vi "Analog Output Engine.vi"(5 "Main Engine Q":refnum<queue>, 7 "TCP Enigine Q":refnum<queue>, 8 "error in":errorcluster, 10 "Engine Name":string, 11 "Varient Data":variant) -> (0 "error out":errorcluster)   [LabVIEW 2024]
doc: "All Rights Reserved © 2017 SyncSols"
uses:
  Controls/Analog Output SM Data Cluster.ctl
  Controls/AIO Command Q Cluster.ctl
  Controls/AO Interface Data Cluster.ctl
  Controls/AO Channel Configuration Cluster.ctl
  Controls/AO Timing Cluster.ctl
  Main Engine/Controls/Main Engine JSON Command State.ctl
  TCP Engine/Controls/TCP Engine I&O  Interupt Cluster.ctl
  Controls/Analog Output SM Cases.ctl
  Main Engine/Controls/Main Engine Engine No.Options.ctl
  Controls/AO JSON Data Cluster.ctl
  Main Engine/Controls/Main Engine Config Confirmation Cluster.ctl
  <vilib>/DAQmx/write.llb/DAQmx Write (Analog 1D Wfm NChan NSamp).vi
  <vilib>/DAQmx/create/channels.llb/DAQmx Create Channel (AO-Voltage-Basic).vi
  <vilib>/DAQmx/create/channels.llb/DAQmx Create Channel (AO-Current-Basic).vi
  <vilib>/DAQmx/configure/timing.llb/DAQmx Timing (Sample Clock).vi
  <vilib>/DAQmx/miscellaneous.llb/DAQmx Fill In Error Info.vi
  TCP Engine/TCP Engine.lvlib
  <resource>/objmgr/daqmx.rc
panel:
  in  "Data Cluster":T1={"Main Engine Respons  Q"=refnum, "TCP Engine Response Q"=refnum, "Start Notifier"=refnum, "Stop Notifier"=refnum, "AO Task"="", "Varient Data"=variant(string ""), "Engine Name"="", "Continous Data Generation"=FALSE, " Command Q"=refnum, "Interupt Q"=refnum, "AO Timing"={"samples per channel"=1000, "sample mode"=10178, "Sampling Rate"=1000.0}, "Configuration Data"=[], "Channel names"=[], "6738 Card?"=FALSE, "AO Log File Path"=path ""} {"AO Timing"."sample mode" items=["Finite Samples"=10178, "Continuous Samples"=10123, "Hardware Timed Single Point"=12522]}
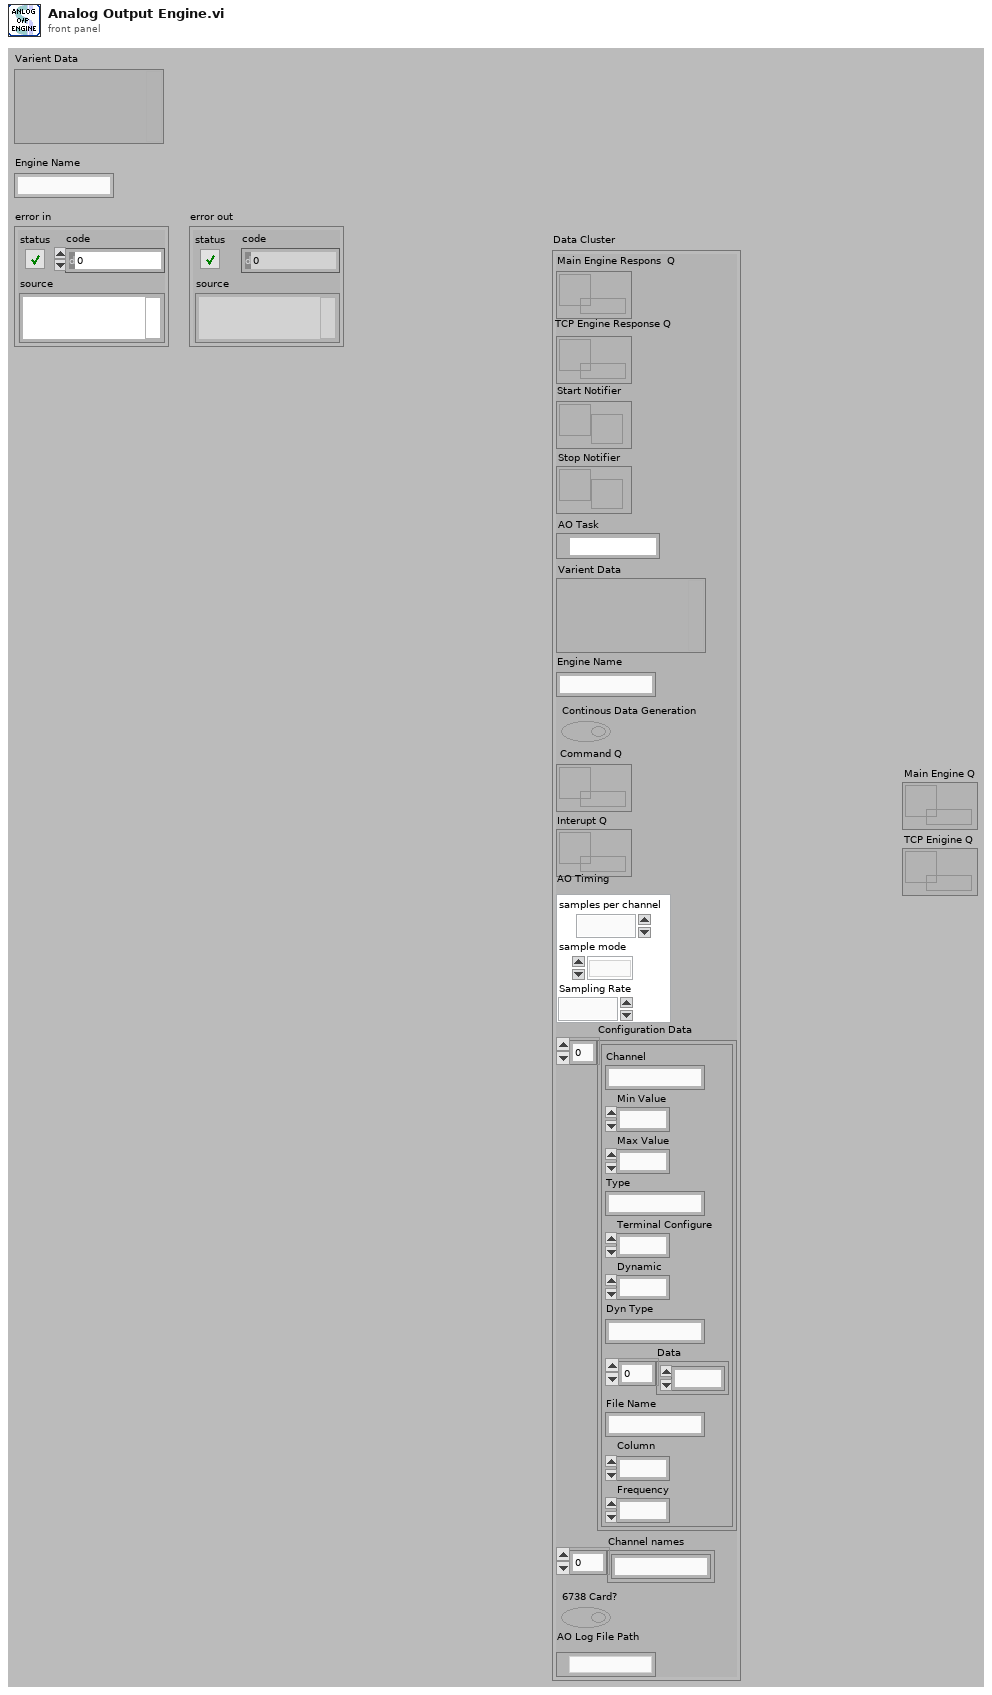
[diagram p1: front panel]
types:
  T1 = typedef "Analog Output SM Data Cluster.ctl" = cluster{"Main Engine Respons  Q":refnum<queue>, "TCP Engine Response Q":refnum<queue>, "Start Notifier":refnum<notifier>, "Stop Notifier":refnum<notifier>, "AO Task":refnum<k21>, "Varient Data":variant, "Engine Name":string, "Continous Data Generation":bool, " Command Q":refnum<queue>, "Interupt Q":refnum<queue>, "AO Timing":T2, "Configuration Data":T3[], "Channel names":string[], "6738 Card?":bool, "AO Log File Path":path}
  T2 = typedef "AO Timing Cluster.ctl" = cluster{"samples per channel":i32, "sample mode":i32, "Sampling Rate":dbl}
  T3 = typedef "AO Channel Configuration Cluster.ctl" = cluster{"Channel":string, "Min Value":dbl, "Max Value":dbl, "Type":string, "Terminal Configure":u16, "Dynamic":u8, "Dyn Type":string, "Data":dbl[], "File Name":string, "Column":i32, "Frequency":dbl}
  T4 = typedef "Analog Output SM Cases.ctl" = enum16{">Poll", ".........State Machine.........", ">Init", ">Error", ">Exit", "..........Analog Output..........", ">JSON to LV Data", ">Gen Dyn Data", ">Get Command", ">Configure", ">Start", ">Generate", ">Stop"}
  T5 = typedef "TCP Engine.lvlib/TCP Engine I&O  Interupt Cluster.ctl" = cluster{" Stop":bool, "JSON Variant":variant}
  T6 = typedef "AIO Command Q Cluster.ctl" = cluster{"Interface":string, "Interface Data":T7, "Command State":T8}
  T7 = typedef "AO Interface Data Cluster.ctl" = cluster{"Command":string, "SubCmd":string, "Data":T3[], "Timing":T2}
  T8 = typedef "Main Engine JSON Command State.ctl" = enum16{"Configure", "Start", "Exit"}
  T9 = typedef "Main Engine Engine No.Options.ctl" = enum16{"Init", "Update", "Response", "Get"}
  T10 = typedef "AO JSON Data Cluster.ctl" = cluster{"Interface":string, "Interface Data":T7}
  T11 = typedef "Main Engine Config Confirmation Cluster.ctl" = cluster{"Command":string, "Interface":string, "Status":string, "Board":string}
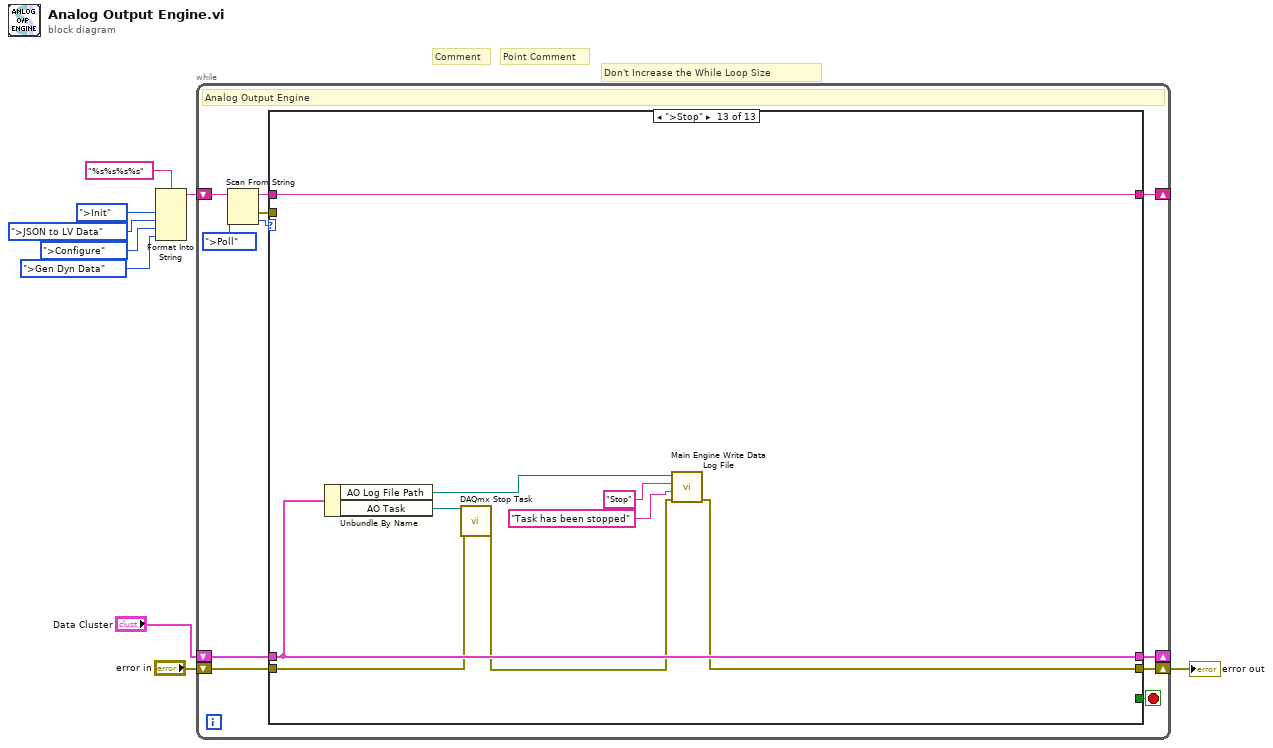
[diagram p0: block diagram]
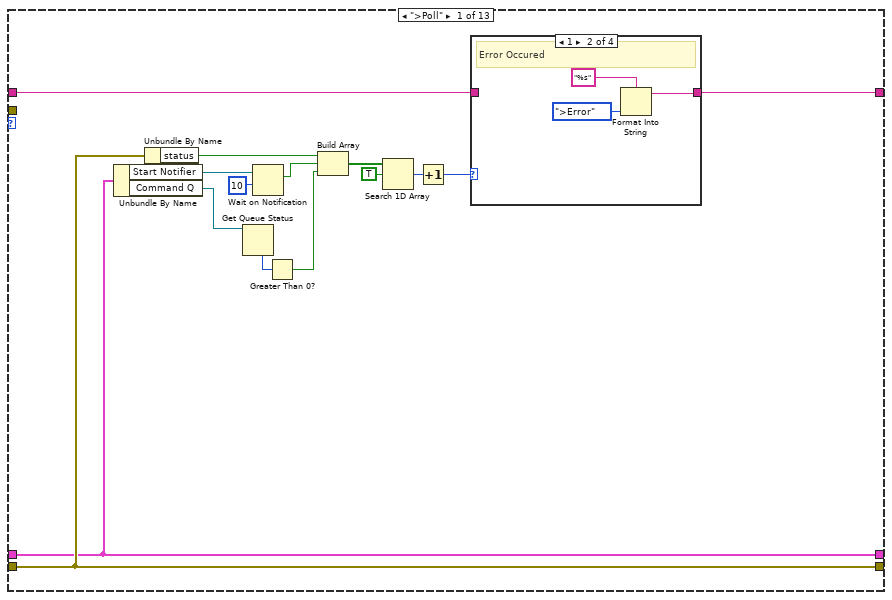
[diagram p2: hidden frame]
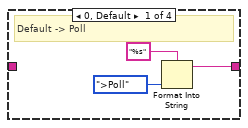
[diagram p3: hidden frame]
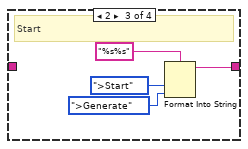
[diagram p4: hidden frame]
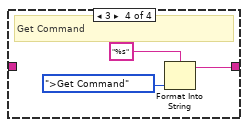
[diagram p5: hidden frame]
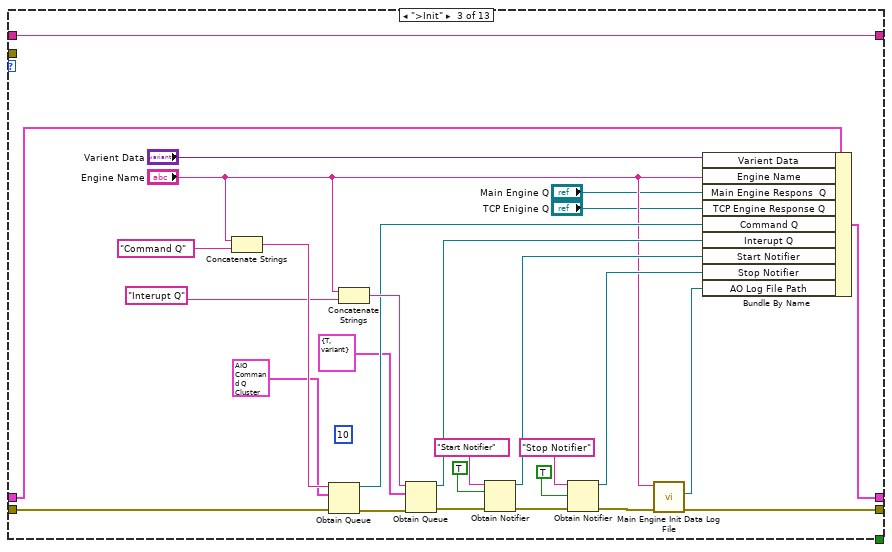
[diagram p7: hidden frame]
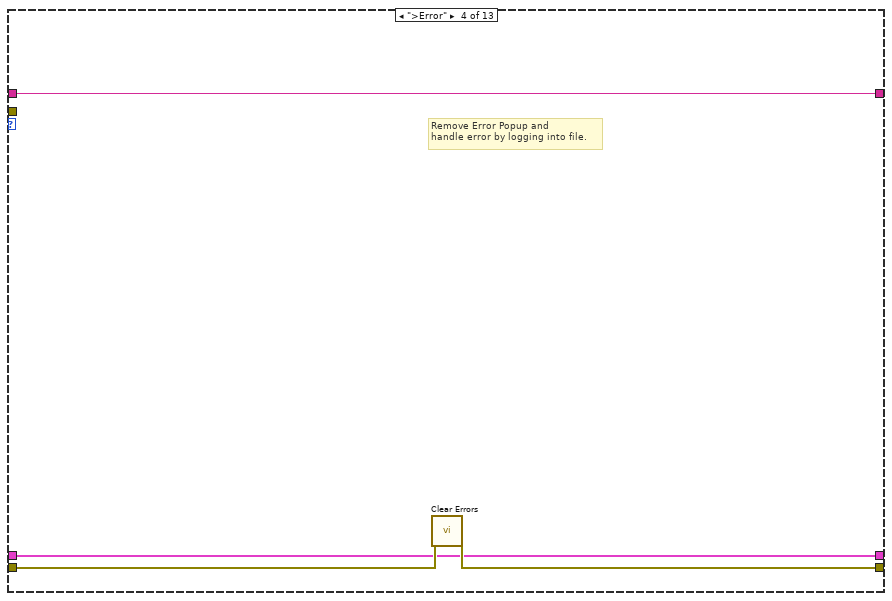
[diagram p8: hidden frame]
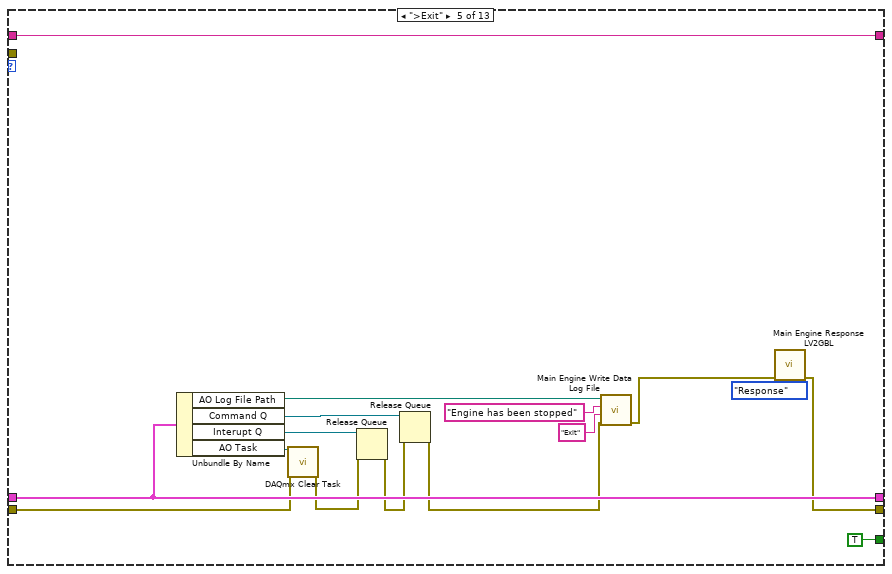
[diagram p9: hidden frame]
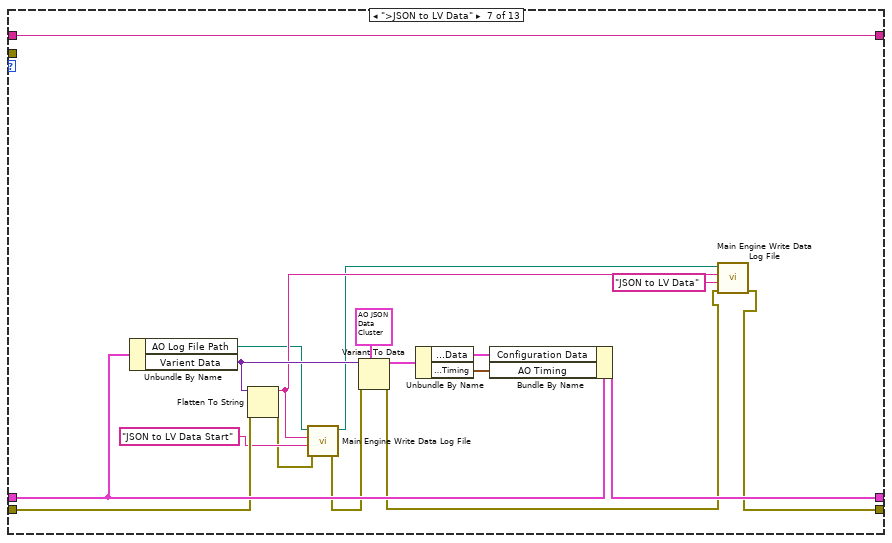
[diagram p11: hidden frame]
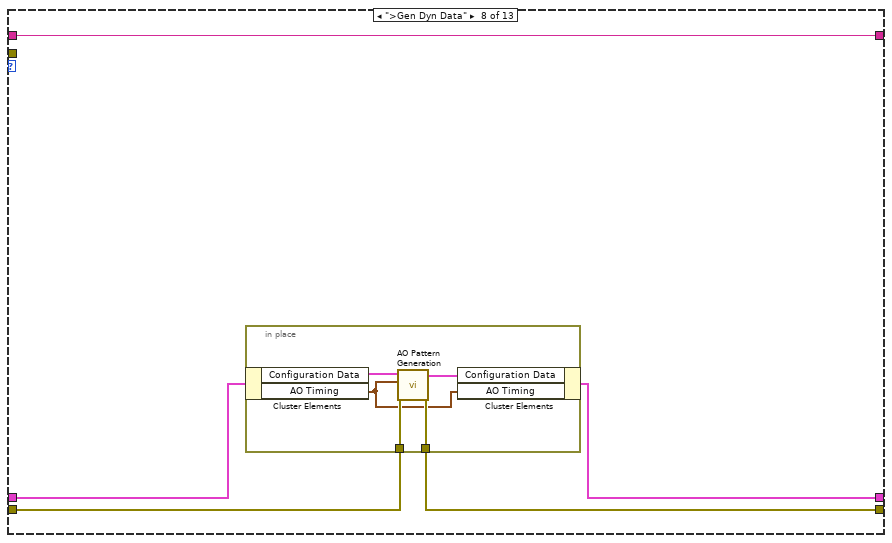
[diagram p12: hidden frame]
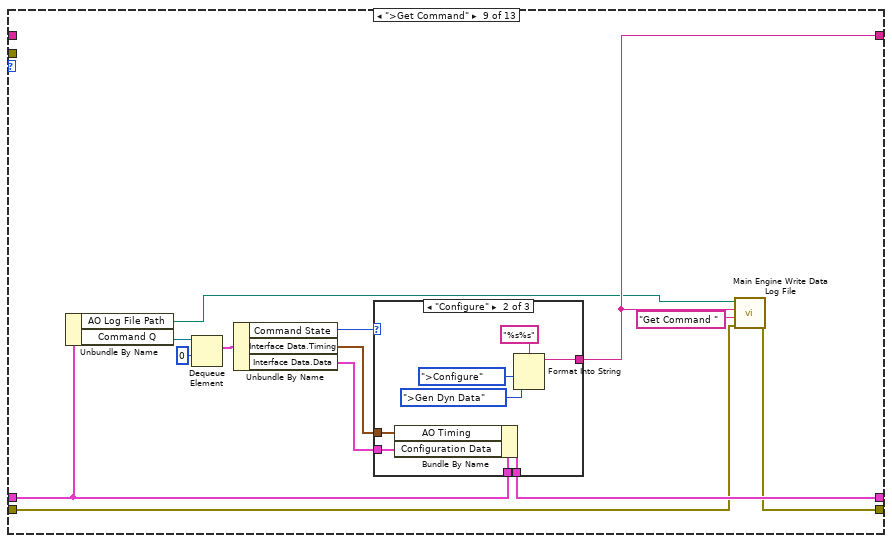
[diagram p13: hidden frame]
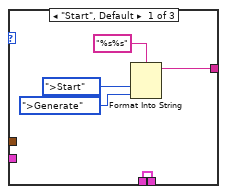
[diagram p14: hidden frame]
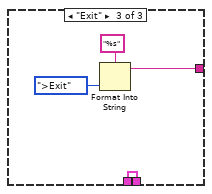
[diagram p15: hidden frame]
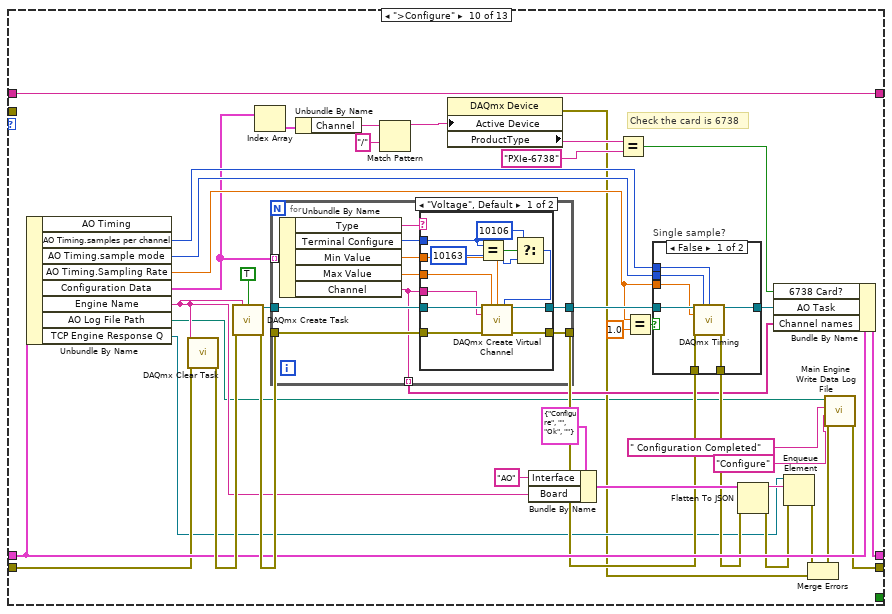
[diagram p16: hidden frame]
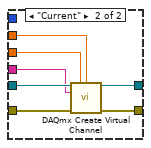
[diagram p18: hidden frame]
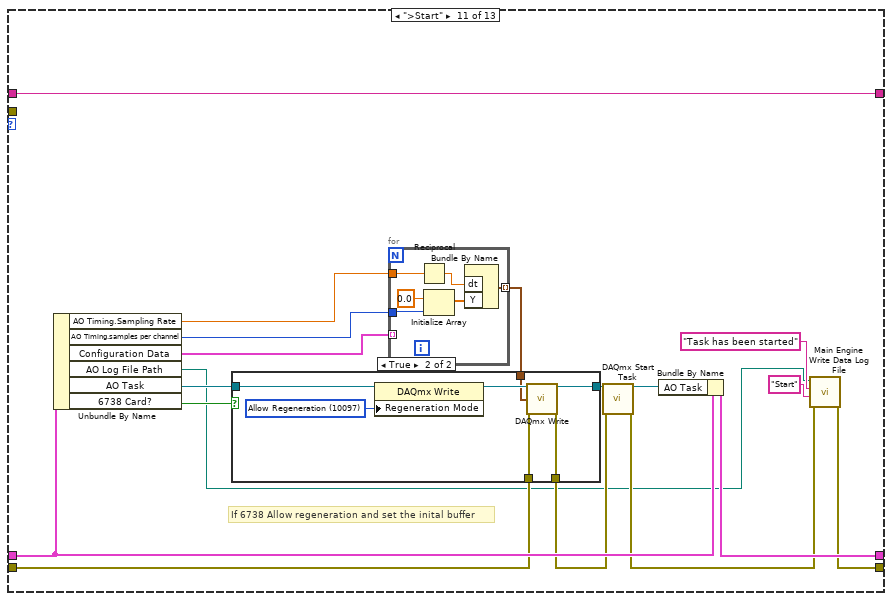
[diagram p19: hidden frame]
diagram:
  # "Don't Increase the While Loop Size"
  # "Point Comment"
  # "Comment"
  n1 = Format Into String(format string="%s%s%s%s", Analog_Output_SM_Cases.">Init" ("SM Cases Options"), Analog_Output_SM_Cases.">JSON to LV Data" ("input 2"), Analog_Output_SM_Cases.">Configure" ("input 3"), Analog_Output_SM_Cases.">Gen Dyn Data" ("input 3")) -> (resulting string=w8:string)  [unwired: 2 in, 1 out]
  n2 = while {
    shift-right: [w15] -> _
    shift-left: w8 -> [w20]
    shift-right: [w13] -> w5
    shift-left: "error in" -> [w14]
    shift-right: [w11] -> _
    shift-left: "Data Cluster" -> [w10]
    stop <- w12 stop-if-true
    # "Analog Output Engine"
    n3 = Scan From String(input string=w20, default 1=Analog_Output_SM_Cases.">Poll" ("SM Cases Options")) -> (remaining string=w16:string, error out=w18:errorcluster, output 1=w17:T4)  [unwired: 3 in, 1 out]
    n4 = case shown="\">Stop\"" w17 {
      tunnel: w18 -> [_ _ _ _ _ _ _ _ _ _ _ _ _]
      tunnel: w16 -> [w35 w51 w79 w83 w99 w102 w120 w125 _ w200 w256 _ w304]
      tunnel: [w34 w51 w79 w83 w99 w102 w120 w125 w135 w200 w256 w292 w304] -> w15
      tunnel: w14 -> [w33 w50 w56 w82 w92 w101 w112 w124 w133 w192 w245 w279 w301]
      tunnel: [w33 w50 w57 w81 w90 w101 w105 w123 w132 w163 w240 w274 w297] -> w13
      tunnel: [_ _ _ _ TRUE _ _ _ _ _ _ _ _] -> w12
      tunnel: [w27 w49 w71 w80 w97 w100 w118 w121 w137 w194 w253 w295 w303] -> w11
      tunnel: w10 -> [w27 w49 w53 w80 w97 w100 w119 w122 w136 w193 w255 w295 w303]
      frame ">Poll" {
        n5 = Unbundle By Name(w27) -> ("Start Notifier"=w26:refnum<notifier>, "Command Q"=w23:refnum<queue>)
        n6 = Unbundle By Name(w33) -> ("status"=w32:bool)
        n7 = Get Queue Status(queue=w23) -> (# elements in queue=w22:i32)  [unwired: 2 in, 7 out]
        n8 = Wait on Notification(notifier=w26, timeout in ms (-1)=10) -> (notification=w25:bool)  [unwired: 2 in, 3 out]
        n9 = Greater Than 0?(x=w22) -> (x > 0?=w21:bool)
        n10 = Build Array(w32, w25, w21) -> (w31:bool[])
        n11 = Search 1D Array(1D array=w31, element=TRUE) -> (index of element=w29:i32)  [unwired: 1 in]
        n12 = Increment(x=w29) -> (x+1=w28:i32)
        n13 = case shown="1" w28 {
          tunnel: w35 -> [_ _ _ _]
          tunnel: [w36 w39 w43 w46] -> w34
          frame 0, Default {
            # "Default -> Poll"
            n14 = Format Into String(format string="%s", Analog_Output_SM_Cases.">Poll" ("SM Cases Options")) -> (resulting string=w36:string)  [unwired: 2 in, 1 out]
          }
          frame 1 {
            # "Error Occured"
            n15 = Format Into String(format string="%s", Analog_Output_SM_Cases.">Error" ("SM Cases Options")) -> (resulting string=w39:string)  [unwired: 2 in, 1 out]
          }
          frame 2 {
            # "Start"
            n16 = Format Into String(format string="%s%s", Analog_Output_SM_Cases.">Start" ("SM Cases Options"), Analog_Output_SM_Cases.">Generate" ("input 2")) -> (resulting string=w43:string)  [unwired: 2 in, 1 out]
          }
          frame 3 {
            # "Get Command"
            n17 = Format Into String(format string="%s", Analog_Output_SM_Cases.">Get Command" ("SM Cases Options")) -> (resulting string=w46:string)  [unwired: 2 in, 1 out]
          }
        }
      }
      frame ".........State Machine........." {
      }
      frame ">Init" {
        (unwired) 10 ("max queue size (-1, unlimited)")
        n18 = Concatenate Strings("Engine Name", "Command Q" ("name (unnamed)")) -> (w66:string)
        n19 = Obtain Queue(name (unnamed)=w66, element data type=T6 {"Interface"="AIO", "Interface Data"={"Command"="Configure", "SubCmd"="AO", "Data"=[], "Timing"={"samples per channel"=1000, "sample mode"=10178, "Sampling Rate"=1000.0}}, "Command State"=enum."Configure"}, error in (no error)=w56) -> (queue out=w62:refnum<queue>, error out=w78:errorcluster)  [unwired: 2 in, 1 out]
        n20 = Concatenate Strings("Engine Name", "Interupt Q" ("name (unnamed)")) -> (w64:string)
        n21 = Obtain Queue(name (unnamed)=w64, element data type=T5 {" Stop"=TRUE, "JSON Variant"=variant(string "")}, error in (no error)=w78) -> (queue out=w60:refnum<queue>, error out=w77:errorcluster)  [unwired: 2 in, 1 out]
        n22 = Obtain Notifier(name (unnamed)="Start Notifier", notification data type=TRUE, error in (no error)=w77) -> (notifier out=w70:refnum<notifier>, error out=w76:errorcluster)  [unwired: 1 in, 1 out]
        n23 = Obtain Notifier(name (unnamed)="Stop Notifier", notification data type=TRUE, error in (no error)=w76) -> (notifier out=w69:refnum<notifier>, error out=w58:errorcluster)  [unwired: 1 in, 1 out]
        n24 = call "Main Engine Init Data Log File.vi"("error in"=w58, "Engine Name"="Engine Name") -> ("error out"=w57:errorcluster, "Log File Path"=w52:path)  [unwired: 8 in]
        n25 = Bundle By Name(cluster=w53, "Varient Data"="Varient Data", "Engine Name"="Engine Name", "Main Engine Respons  Q"="Main Engine Q", "TCP Engine Response Q"="TCP Enigine Q", "Command Q"=w62, "Interupt Q"=w60, "Start Notifier"=w70, "Stop Notifier"=w69, "AO Log File Path"=w52) -> (w71:T1)
      }
      frame ">Error" {
        # "Remove Error Popup and \nhandle error by logging into file."
        n26 = call <vilib>:"Clear Errors.vi"("error in (no error)"=w82) -> ("error out"=w81:errorcluster)  [unwired: 5 in, 1 out]
      }
      frame ">Exit" {
        n27 = Unbundle By Name(w97) -> ("AO Log File Path"=w84:path, "Command Q"=w94:refnum<queue>, "Interupt Q"=w95:refnum<queue>, "AO Task"=w91:refnum<k21>)
        n28 = call <vilib>:"DAQmx Clear Task.vi"("task in"=w91, "error in"=w92) -> ("error out"=w93:errorcluster)  [unwired: 13 in]
        n29 = Release Queue(queue=w95, error in (no error)=w93) -> (error out=w96:errorcluster)  [unwired: 1 in, 2 out]
        n30 = Release Queue(queue=w94, error in (no error)=w96) -> (error out=w86:errorcluster)  [unwired: 1 in, 2 out]
        n31 = call "Main Engine Write Data Log File.vi"("error in"=w86, "State"="Exit", "Input Data"="Engine has been stopped" ("State"), "Log file path In"=w84) -> ("error out"=w85:errorcluster)  [unwired: 6 in, 1 out]
        n32 = call "Main Engine Response LV2GBL.vi"("Options"=Main_Engine_Engine_No.Options."Response", "error in"=w85) -> ("error out"=w90:errorcluster)  [unwired: 7 in, 2 out]
      }
      frame "..........Analog Output.........." {
      }
      frame ">JSON to LV Data" {
        n33 = Unbundle By Name(w119) -> ("AO Log File Path"=w104:path, "Varient Data"=w115:variant)
        n34 = Flatten To String(anything=w115, error in (no error)=w112) -> (data string=w108:string, error out=w110:errorcluster)  [unwired: 2 in, 1 out]
        n35 = call "Main Engine Write Data Log File.vi"("error in"=w110, "State"="JSON to LV Data Start", "Input Data"=w108, "Log file path In"=w104) -> ("error out"=w109:errorcluster, "Log File Path Out"=w103:path)  [unwired: 6 in]
        n36 = Variant To Data(error in=w109, type=T10 {"Interface"="AIO", "Interface Data"={"Command"="Configure", "SubCmd"="AO", "Data"=[], "Timing"={"samples per channel"=1000, "sample mode"=10178, "Sampling Rate"=1000.0}}} ("AO JSON Data Cluster"), Variant=w115) -> (data=w117:T10, error out=w106:errorcluster)
        n37 = Unbundle By Name(w117) -> ("Interface Data.Data"=w114:T3[], "Interface Data.Timing"=w113:T2)
        n38 = Bundle By Name(cluster=w119, "Configuration Data"=w114, "AO Timing"=w113) -> (w118:T1)
        n39 = call "Main Engine Write Data Log File.vi"("error in"=w106, "State"="JSON to LV Data", "Input Data"=w108, "Log file path In"=w103) -> ("error out"=w105:errorcluster)  [unwired: 6 in, 1 out]
      }
      frame ">Gen Dyn Data" {
        n40 = in-place {
          in-place-border: w124 -> [w130]
          in-place-border: [w129] -> w123
          n41 = in-place-cluster #1(w122) -> ("Configuration Data"=w128:T3[], "AO Timing"=w126:T2)
          n42 = call "AO Pattern Generation.vi"("error in"=w130, "Timing"=w126, "Config"=w128) -> ("error out"=w129:errorcluster, "Config"=w127:T3[])  [unwired: 7 in]
          n43 = in-place-cluster #1("Configuration Data"=w127, "AO Timing"=w126) -> (w121:T1)
        }
      }
      frame ">Get Command" {
        n44 = Unbundle By Name(w136) -> ("AO Log File Path"=w131:path, "Command Q"=w143:refnum<queue>)
        n45 = Dequeue Element(queue=w143, timeout in ms (-1)=0) -> (element=w141:T6)  [unwired: 1 in, 3 out]
        n46 = Unbundle By Name(w141) -> ("Command State"=w140:T8, "Interface Data.Timing"=w139:T2, "Interface Data.Data"=w138:T3[])
        n47 = case shown="\"Configure\"" w140 {
          tunnel: [w146 w154 w158] -> w135
          tunnel: w139 -> [_ w153 _]
          tunnel: w138 -> [_ w152 _]
          tunnel: w136 -> [w144 w151 w157]
          tunnel: [w144 w150 w157] -> w137
          frame "Start", Default {
            n48 = Format Into String(format string="%s%s", Analog_Output_SM_Cases.">Start" ("SM Cases Options"), Analog_Output_SM_Cases.">Generate" ("input 2")) -> (resulting string=w146:string)  [unwired: 2 in, 1 out]
          }
          frame "Configure" {
            n49 = Bundle By Name(cluster=w151, "AO Timing"=w153, "Configuration Data"=w152) -> (w150:T1)
            n50 = Format Into String(format string="%s%s", Analog_Output_SM_Cases.">Configure" ("SM Cases Options"), Analog_Output_SM_Cases.">Gen Dyn Data" ("SM Cases Options")) -> (resulting string=w154:string)  [unwired: 2 in, 1 out]
          }
          frame "Exit" {
            n51 = Format Into String(format string="%s", Analog_Output_SM_Cases.">Exit" ("SM Cases Options")) -> (resulting string=w158:string)  [unwired: 2 in, 1 out]
          }
        }
        n52 = call "Main Engine Write Data Log File.vi"("error in"=w133, "State"="Get Command ", "Input Data"=w135, "Log file path In"=w131) -> ("error out"=w132:errorcluster)  [unwired: 6 in, 1 out]
      }
      frame ">Configure" {
        # "Check the card is 6738"
        n53 = Unbundle By Name(w193) -> ("AO Timing.samples per channel"=w191:i32, "AO Timing.sample mode"=w190:i32, "AO Timing.Sampling Rate"=w188:dbl, "Configuration Data"=w177:T3[], "Engine Name"=w168:string, "AO Log File Path"=w161:path, "TCP Engine Response Q"=w179:refnum<queue>)  [unwired: 1 out]
        n54 = call <vilib>:"DAQmx Clear Task.vi"("task in"=w168, "error in"=w192) -> ("error out"=w199:errorcluster)  [unwired: 13 in]
        n55 = call <vilib>:"DAQmx Create Task.vi"("new task name"=w168, "auto cleanup"=TRUE, "error in"=w199) -> ("task out"=w197:refnum<k21>, "error out"=w198:errorcluster)  [unwired: 11 in]
        n56 = Index Array(array=w177) -> (element=w176:T3)  [unwired: 1 in]
        n57 = for {
          tunnel: w198 -> [w219]
          tunnel: [w218] -> w182
          tunnel: w197 -> [w217]
          tunnel: [w216] -> w196
          tunnel: w177 -> [w215] mode=indexing
          tunnel: [w210] -> w178 mode=indexing
          n58 = Unbundle By Name(w215) -> ("Type"=w212:string, "Terminal Configure"=w211:u16, "Min Value"=w214:dbl, "Max Value"=w213:dbl, "Channel"=w210:string)
          n59 = case shown="\"Voltage\", Default" w212 {
            tunnel: w219 -> [w231 w238]
            tunnel: [w230 w237] -> w218
            tunnel: w217 -> [w229 w236]
            tunnel: [w228 w235] -> w216
            tunnel: w210 -> [w227 w234]
            tunnel: w214 -> [w226 w233]
            tunnel: w213 -> [w225 w232]
            tunnel: w211 -> [w222 _]
            frame "Voltage", Default {
              n60 = Equal?(x=w222, y=u16 10163) -> (x = y?=w223:bool)
              n61 = Select(t=u16 10106, s=w223, f=w222) -> (s? t:f=w220:u16)
              n62 = call-poly <vilib>:"DAQmx Create Virtual Channel.vi"("task in"=w229, "maximum value"=w225, "minimum value"=w226, "output terminal configuration"=w220, "physical channels"=w227, "error in"=w231) -> ("task out"=w228:refnum<k21>, "error out"=w230:errorcluster)  [unwired: 8 in]
            }
            frame "Current" {
              n63 = call-poly <vilib>:"DAQmx Create Virtual Channel.vi"("task in"=w236, "maximum value"=w232, "minimum value"=w233, "physical channels"=w234, "error in"=w238) -> ("task out"=w235:refnum<k21>, "error out"=w237:errorcluster)  [unwired: 9 in]
            }
          }
        }
        n64 = Unbundle By Name(w176) -> ("Channel"=w175:string)
        n65 = Match Pattern(string=w175, regular expression="/") -> (before substring=w173:string)  [unwired: 1 in, 3 out]
        n66 = property class="DAQmx Device"("Active Device"=w173) -> (error out=w169:errorcluster, "ProductType"=w172:string)  [unwired: 2 in, 1 out]
        n67 = Bundle By Name(cluster=T11 {"Command"="Configure", "Interface"="", "Status"="Ok", "Board"=""} ("Config Confirmation"), "Interface"="AO" ("SubCmd"), "Board"=w168) -> (w186:T11)
        n68 = Equal?(x=w172, y="PXIe-6738") -> (x = y?=w170:bool)
        n69 = Equal?(x=w188, y=1.0) -> (x = y?=w187:bool)
        n70 = case "Single sample?" shown="False" w187 {
          tunnel: w182 -> [w207 w208]
          tunnel: w196 -> [w206 w209]
          tunnel: [w205 w209] -> w195
          tunnel: w191 -> [w204 _]
          tunnel: w190 -> [w203 _]
          tunnel: w188 -> [w202 _]
          tunnel: [w201 w208] -> w181
          frame False {
            n71 = call-poly <vilib>:"DAQmx Timing.vi"("task/channels in"=w206, "sample mode"=w203, "samples per channel"=w204, "rate"=w202, "error in"=w207) -> ("task out"=w205:refnum<k21>, "error out"=w201:errorcluster)  [unwired: 9 in]
          }
          frame True {
          }
        }
        n72 = Flatten To JSON(anything=w186, error in (no error)=w181) -> (JSON string=w185:string, 11:w183:errorcluster)  [unwired: 1 in]
        n73 = Bundle By Name(cluster=w193, "6738 Card?"=w170, "AO Task"=w195, "Channel names"=w178) -> (w194:T1)
        n74 = Enqueue Element(queue=w179, element=w185, error in (no error)=w183) -> (error out=w180:errorcluster)  [unwired: 1 in, 2 out]
        n75 = Merge Errors(w180, w169) -> (w164:errorcluster)
        n76 = call "Main Engine Write Data Log File.vi"("error in"=w164, "State"="Configure", "Input Data"=" Configuration Completed", "Log file path In"=w161) -> ("error out"=w163:errorcluster)  [unwired: 6 in, 1 out]
      }
      frame ">Start" {
        # "If 6738 Allow regeneration and set the inital buffer"
        n77 = Unbundle By Name(w255) -> ("AO Timing.Sampling Rate"=w249:dbl, "AO Timing.samples per channel"=w250:i32, "Configuration Data"=w251:T3[], "AO Log File Path"=w239:path, "AO Task"=w252:refnum<k21>, "6738 Card?"=w244:bool)
        n78 = for {
          tunnel: w251 -> [_] mode=indexing
          tunnel: w250 -> [w271]
          tunnel: w249 -> [w269]
          tunnel: [w268] -> w246 mode=indexing
          n79 = Reciprocal(x=w269) -> (1/x=w270:dbl)
          n80 = Initialize Array(0.0 ("element"), w271) -> (w266:dbl[])
          n81 = Bundle By Name("dt"=w270, "Y"=w266) -> (w268:waveform(dbl))  [unwired: 1 in]
        }
        n82 = case shown="True" w244 {
          tunnel: w252 -> [w257 w264]
          tunnel: [w258 w263] -> w248
          tunnel: [w257 w262] -> w247
          tunnel: w246 -> [_ w260]
          tunnel: w245 -> [w258 w259]
          frame False {
          }
          frame True {
            w265 = 10097 items=["Allow Regeneration"=10097, "Do Not Allow Regeneration"=10158] ("RegenMode")
            n83 = property class="DAQmx Write"(reference=w264, "Regeneration Mode"=w265) -> (reference out=w261:refnum<k21>)  [unwired: 1 in, 1 out]
            n84 = call-poly <vilib>:"DAQmx Write.vi"("task/channels in"=w261, "data"=w260, "error in"=w259) -> ("task out"=w262:refnum<k21>, "error out"=w263:errorcluster)  [unwired: 10 in, 1 out]
          }
        }
        n85 = call <vilib>:"DAQmx Start Task.vi"("task/channels in"=w247, "error in"=w248) -> ("task out"=w254:refnum<k21>, "error out"=w241:errorcluster)  [unwired: 12 in]
        n86 = Bundle By Name(cluster=w255, "AO Task"=w254) -> (w253:T1)
        n87 = call "Main Engine Write Data Log File.vi"("error in"=w241, "State"="Start", "Input Data"="Task has been started" ("State"), "Log file path In"=w239) -> ("error out"=w240:errorcluster)  [unwired: 6 in, 1 out]
      }
      frame ">Generate" {
        n88 = Unbundle By Name(w295) -> ("AO Timing"=w285:T2, "6738 Card?"=w282:bool, "AO Task"=w288:refnum<k21>, "Interupt Q"=w289:refnum<queue>, "Main Engine Respons  Q"=w290:refnum<queue>, "Stop Notifier"=w291:refnum<notifier>, "AO Log File Path"=w273:path, "Configuration Data"=w284:T3[])
        n89 = call "Main Engine Write Data Log File.vi"("error in"=w279, "State"="Generate", "Input Data"="Data Generation Started", "Log file path In"=w273) -> ("error out"=w278:errorcluster, "Log File Path Out"=w272:path)  [unwired: 6 in]
        n90 = call "Analog Output Data Generation.vi"("AO Timing"=w285, "Configuration Data"=w284, "6738 Card?"=w282, "Path"=w273, "AO Task"=w288, "error in"=w278, "Stop Notifier"=w291, "Main Engine Respons  Q"=w290, "Interupt Q"=w289) -> ("error out"=w275:errorcluster, "All Stop"=w283:bool)  [unwired: 1 in]
        n91 = Select(t="Stopped By AO stop", s=w283, f="Stopped By All stop") -> (s? t:f=w277:string)
        n92 = Format Into String(format string="%s", Analog_Output_SM_Cases.">Stop" ("SM Cases Options")) -> (resulting string=w292:string)  [unwired: 2 in, 1 out]
        n93 = call "Main Engine Write Data Log File.vi"("error in"=w275, "State"="Generate", "Input Data"=w277, "Log file path In"=w272) -> ("error out"=w274:errorcluster)  [unwired: 6 in, 1 out]
      }
      frame ">Stop" {
        n94 = Unbundle By Name(w303) -> ("AO Log File Path"=w296:path, "AO Task"=w302:refnum<k21>)
        n95 = call <vilib>:"DAQmx Stop Task.vi"("task/channels in"=w302, "error in"=w301) -> ("error out"=w298:errorcluster)  [unwired: 12 in, 1 out]
        n96 = call "Main Engine Write Data Log File.vi"("error in"=w298, "State"="Task has been stopped", "Input Data"="Stop" ("State"), "Log file path In"=w296) -> ("error out"=w297:errorcluster)  [unwired: 6 in, 1 out]
      }
    }
  }
  "error out" <- w5
